vi "get-Binary-Image.vi"() -> ()   [LabVIEW 2024]
uses:
  <vilib>/vision/NI_Vision_Development_Module.lvlib
panel:
  out "Invertida-Threshold":T1(plugin-control)
  out "Invertida-FillHoles":T1(plugin-control)
  out "Invertida-BorderRejected":T1(plugin-control)
  out "BorderRejected":T1(plugin-control)
  out "FillHoles":T1(plugin-control)
  out "Threshold":T1(plugin-control)
  in  "Range":cluster{"Lower value":sgl, "Upper value":sgl}={"Lower value"=128.0, "Upper value"=255.0} {"Upper value" format="%.2f"; "Lower value" format="%.2f"}
  out "Waveform Graph":T2(graph)
  out "Gray Image":T1(plugin-control)
  in  "GRABAR":bool
  in  "stop":bool
  out "Full Image":T1(plugin-control)
  out "error out":errorcluster
  out "Ojo":T1(plugin-control)
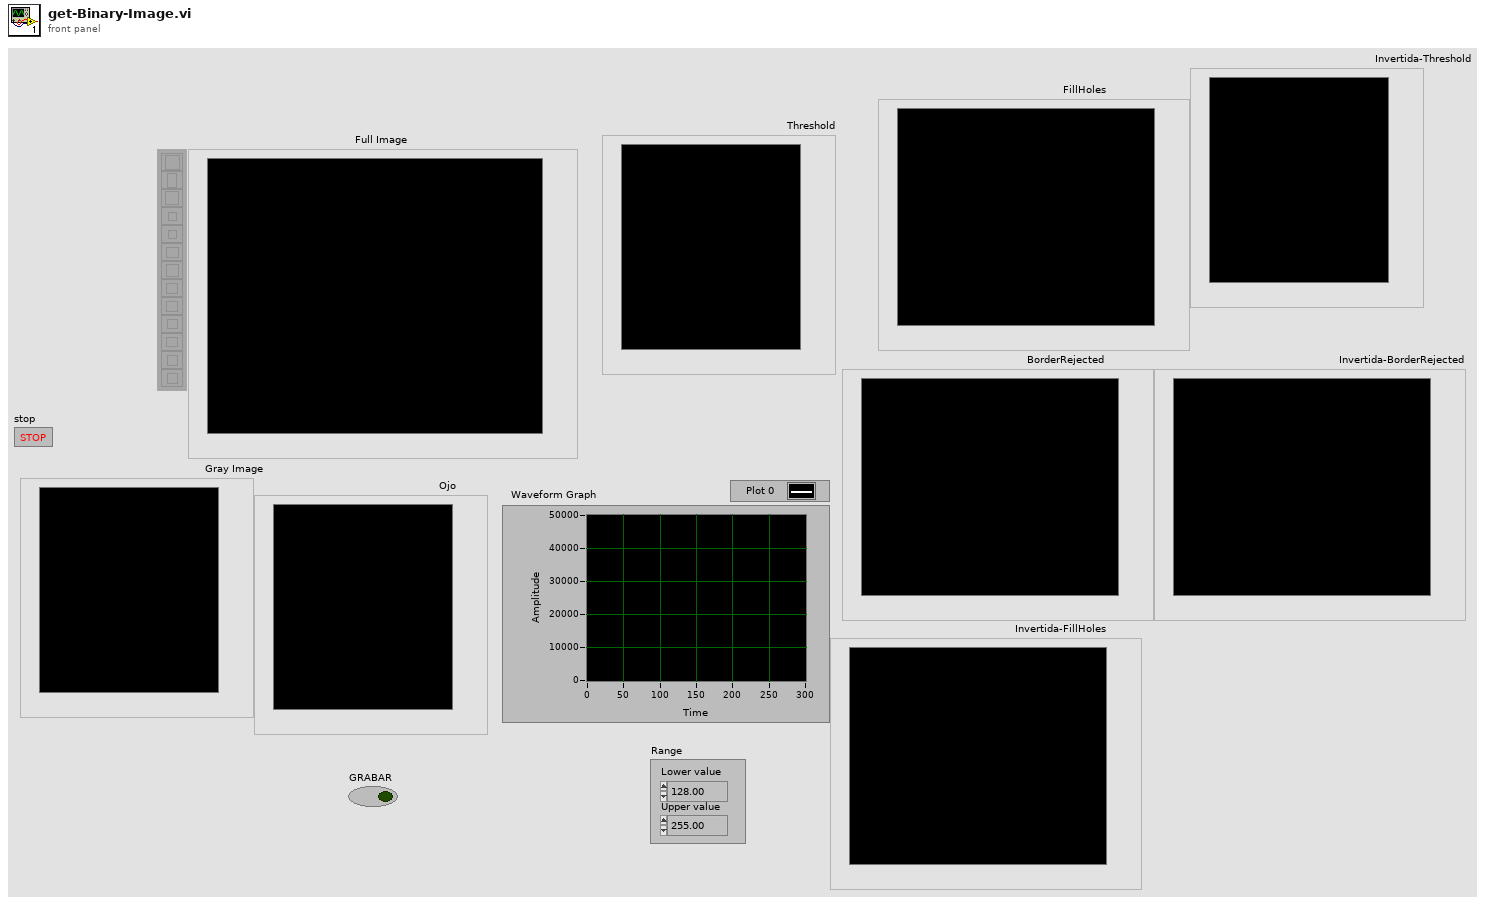
[diagram p1: front panel]
types:
  T1 = typedef "IMAQ Image.ctl" = refnum<image>
  T2 = cluster{"Starting Value":sgl, "Incremental Value":sgl, "Histogram":u32[]}
  T3 = typedef "Image Type" = u32
  T4 = typedef "IMAQ AVI2 Refnum.ctl" = refnum<k20>
  T5 = cluster{"Global Rectangle":i32[], "Contours":cluster{"Contour Type":u32, "ROI Type":u32, "Points":i32[]}[]}
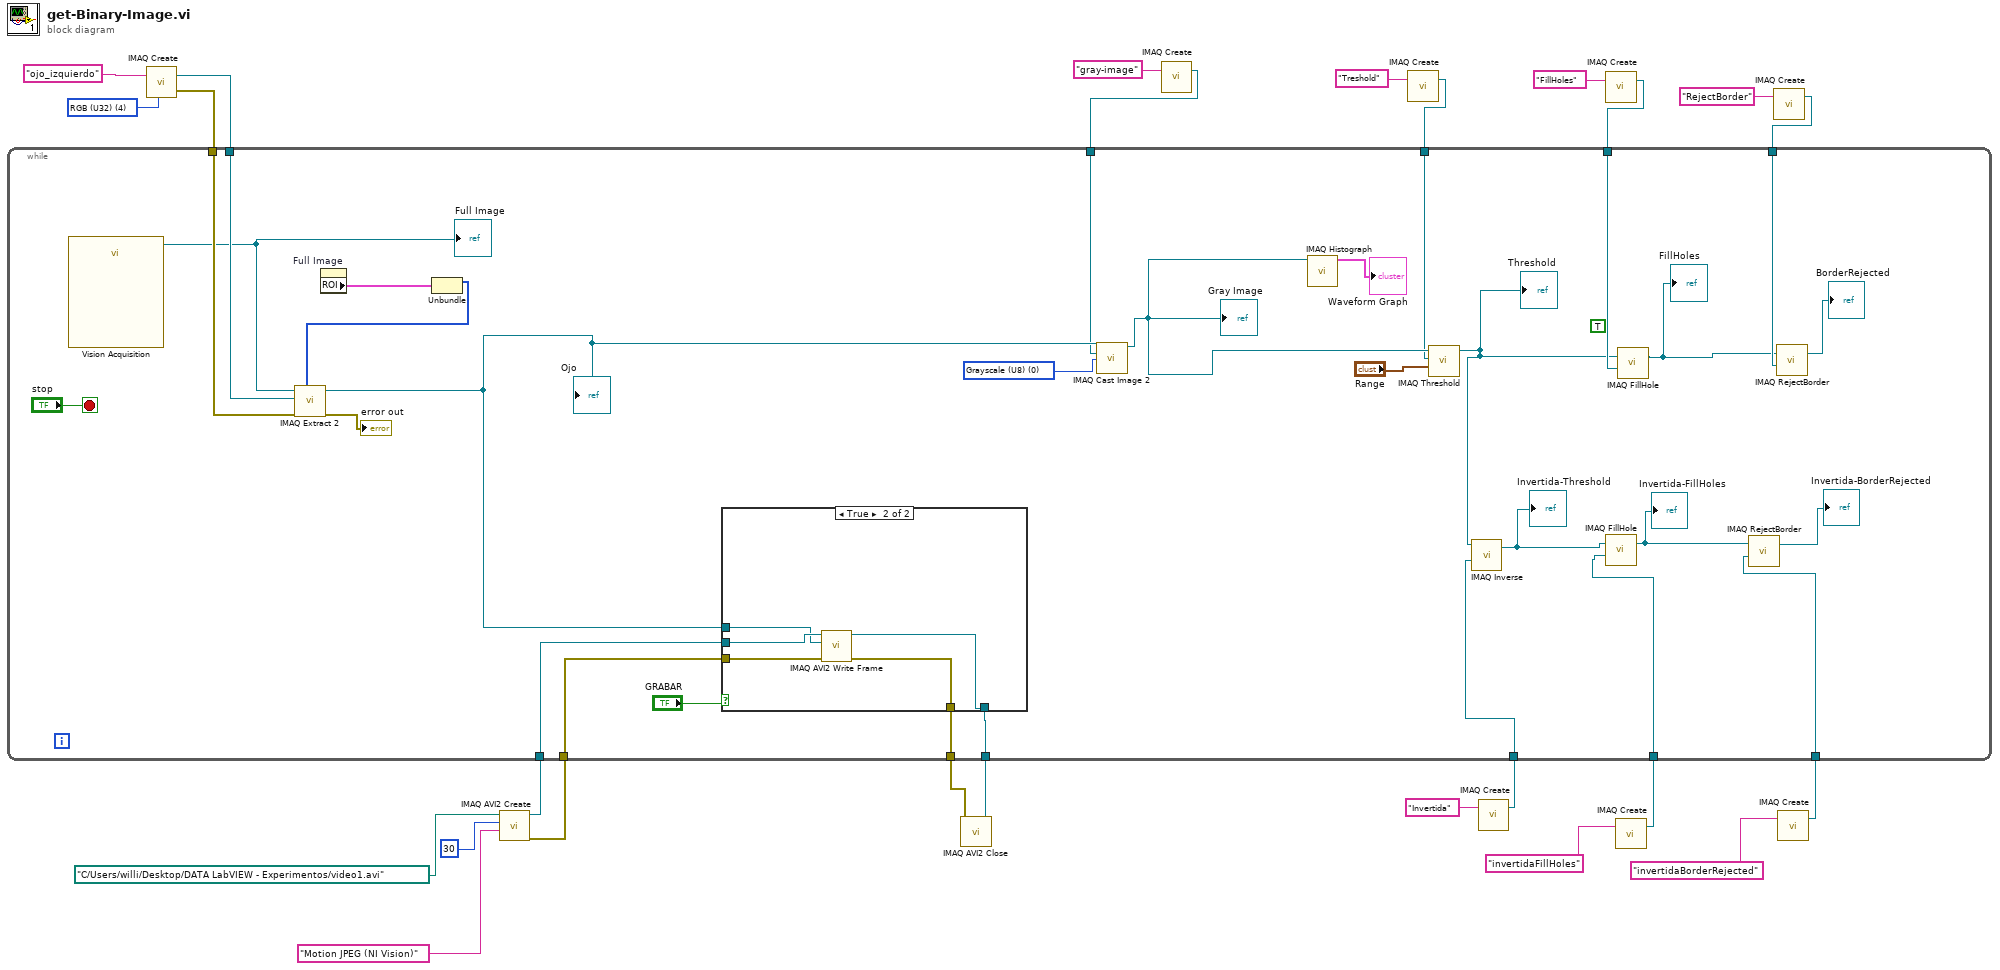
[diagram p0: block diagram]
diagram:
  w24 = T3 4 items=["Grayscale (U8)", "Grayscale (I16)", "Grayscale (SGL)", "Complex (CSG)", "RGB (U32)", "HSL (U32)", "RGB (U64)", "Grayscale (U16)"] ("Image Type")
  n1 = call "IMAQ Create"("Image Name"="ojo_izquierdo", "Image Type"=w24) -> ("New Image"=w22:T1, "error out"=w23:errorcluster)  [unwired: 3 in]
  n2 = call "IMAQ AVI2 Create"("Codec"="Motion JPEG (NI Vision)", "Frames Per Second"=u32 30, "AVI Path"=path "C:/Users/willi/Desktop/DATA LabVIEW - Experimentos/video1.avi") -> ("error out"=w18:errorcluster, "AVI Refnum"=w17:T4)  [unwired: 7 in]
  n3 = call "IMAQ Create"("Image Name"="gray-image") -> ("New Image"=w13:T1)  [unwired: 4 in, 1 out]
  n4 = call "IMAQ Create"("Image Name"="Treshold") -> ("New Image"=w11:T1)  [unwired: 4 in, 1 out]
  n5 = call "IMAQ Create"("Image Name"="Invertida") -> ("New Image"=w7:T1)  [unwired: 4 in, 1 out]
  n6 = call "IMAQ Create"("Image Name"="FillHoles") -> ("New Image"=w9:T1)  [unwired: 4 in, 1 out]
  n7 = call "IMAQ Create"("Image Name"="invertidaFillHoles") -> ("New Image"=w5:T1)  [unwired: 4 in, 1 out]
  n8 = call "IMAQ Create"("Image Name"="RejectBorder") -> ("New Image"=w3:T1)  [unwired: 4 in, 1 out]
  n9 = call "IMAQ Create"("Image Name"="invertidaBorderRejected") -> ("New Image"=w1:T1)  [unwired: 4 in, 1 out]
  n10 = while {
    tunnel: w23 -> [w54]
    tunnel: w22 -> [w53]
    tunnel: w18 -> [w47]
    tunnel: w17 -> [w46]
    tunnel: [w45] -> w16
    tunnel: [w44] -> w15
    tunnel: w13 -> [w42]
    tunnel: w11 -> [w37]
    tunnel: w9 -> [w35]
    tunnel: w7 -> [w36]
    tunnel: w5 -> [w33]
    tunnel: w3 -> [w34]
    tunnel: w1 -> [w32]
    stop <- "stop" stop-if-true
    (unwired) TRUE ("Connectivity 4/8 (8)")
    w41 = T3 0 items=["Grayscale (U8)", "Grayscale (I16)", "Grayscale (SGL)", "Complex (CSG)", "RGB (U32)", "HSL (U32)", "RGB (U64)", "Grayscale (U16)"] ("Image Type")
    n11 = call "Vision Acquisition"() -> ("Image Out"=w49:T1)  [unwired: 25 in, 2 out]
    "Full Image" <- w49
    n12 = property on="Full Image" class="ImageControl"() -> ("ROI"=w52:T5)  [unwired: 2 in, 2 out]
    n13 = Unbundle "Unbundle"(w52) -> ("Global Rectangle"=w51:i32[])  [unwired: 1 out]
    n14 = call "IMAQ Extract 2"("Optional Rectangle"=w51, "error in (no error)"=w54, "Image Dst"=w53, "Image Src"=w49) -> ("error out"=→"error out":errorcluster, "Image Dst Out"=w43:T1)  [unwired: 6 in]
    "Ojo" <- w43
    n15 = case shown="True" "GRABAR" {
      tunnel: w46 -> [w57 w62]
      tunnel: w47 -> [w56 w61]
      tunnel: [w56 w60] -> w45
      tunnel: [w57 w59] -> w44
      tunnel: w43 -> [_ w58]
      frame False {
      }
      frame True {
        n16 = call "IMAQ AVI2 Write Frame"("error in (no error)"=w61, "Image"=w58, "AVI Refnum"=w62) -> ("error out"=w60:errorcluster, "AVI Refnum (duplicate)"=w59:T4)  [unwired: 6 in, 1 out]
      }
    }
    n17 = call "IMAQ Cast Image 2"("Image Src"=w43, "Image Dst"=w42, "Image Type"=w41) -> ("Image Dst Out"=w38:T1)  [unwired: 11 in, 1 out]
    "Gray Image" <- w38
    n18 = call "IMAQ Histograph"("Image"=w38) -> ("Histogram Graph"=→"Waveform Graph":T2)  [unwired: 7 in, 3 out]
    n19 = call "IMAQ Threshold"("Range"="Range", "Image Dst"=w37, "Image Src"=w38) -> ("Image Dst Out"=w27:T1)  [unwired: 7 in, 1 out]
    "Threshold" <- w27
    n20 = call "IMAQ Inverse"("Image Dst"=w36, "Image Src"=w27) -> ("Image Dst Out"=w29:T1)  [unwired: 8 in, 1 out]
    "Invertida-Threshold" <- w29
    n21 = call "IMAQ FillHole"("Image Dst"=w33, "Image Src"=w29) -> ("Image Dst Out"=w30:T1)  [unwired: 4 in, 1 out]
    "Invertida-FillHoles" <- w30
    n22 = call "IMAQ FillHole"("Image Dst"=w35, "Image Src"=w27) -> ("Image Dst Out"=w26:T1)  [unwired: 4 in, 1 out]
    "FillHoles" <- w26
    n23 = call "IMAQ RejectBorder"("Image Dst"=w32, "Image Src"=w30) -> ("Image Dst Out"=→"Invertida-BorderRejected":T1)  [unwired: 4 in, 1 out]
    n24 = call "IMAQ RejectBorder"("Image Dst"=w34, "Image Src"=w26) -> ("Image Dst Out"=→"BorderRejected":T1)  [unwired: 4 in, 1 out]
  }
  n25 = call "IMAQ AVI2 Close"("error in (no error)"=w16, "AVI Refnum"=w15) -> ()  [unwired: 9 in, 1 out]
